vi "get desired labview version.vi"(11 "command line arguments":T1) -> (1 "exe path":path, 2 "lv path specified":bool, 3 "lv version":dbl)   [LabVIEW 2019]
uses:
  arguments.ctl
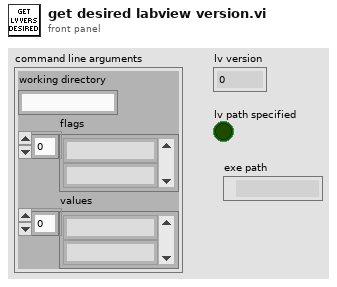
[diagram p1: front panel]
types:
  T1 = typedef "arguments.ctl" = cluster{"working directory":string, "flags":string[], "values":string[]}
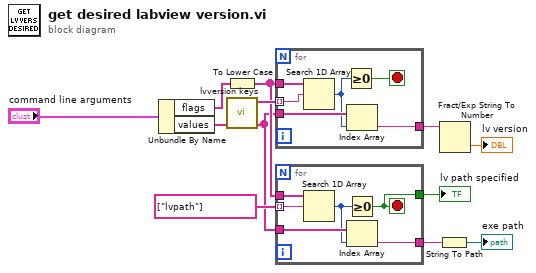
[diagram p0: block diagram]
diagram:
  n1 = Unbundle By Name("command line arguments") -> ("flags"=w7:string[], "values"=w4:string[])
  n2 = To Lower Case(string=w7) -> (all lower case string=w6:string[])
  n3 = call "lvversion keys.vi"() -> ("lv version keys"=w9:string[])  [unwired: 11 in]
  n4 = for {
    tunnel: w6 -> [w17]
    tunnel: w4 -> [w15]
    tunnel: w9 -> [w16] mode=indexing
    tunnel: [w14] -> w8
    stop <- w12 stop-if-true
    n5 = Search 1D Array(1D array=w17, element=w16) -> (index of element=w13:i32)  [unwired: 1 in]
    n6 = Greater Or Equal To 0?(x=w13) -> (x >= 0?=w12:bool)
    n7 = Index Array(array=w15, index=w13) -> (element=w14:string)
  }
  n8 = for {
    tunnel: w6 -> [w23]
    tunnel: w4 -> [w21]
    tunnel: string[] ["lvpath"] ("lv version keys") -> [w22] mode=indexing
    tunnel: [w20] -> w3
    tunnel: [w18] -> w1
    stop <- w18 stop-if-true
    n9 = Search 1D Array(1D array=w23, element=w22) -> (index of element=w19:i32)  [unwired: 1 in]
    n10 = Greater Or Equal To 0?(x=w19) -> (x >= 0?=w18:bool)
    n11 = Index Array(array=w21, index=w19) -> (element=w20:string)
  }
  "lv path specified" <- w1
  n12 = String To Path(string=w3) -> (path=→"exe path":path)
  n13 = Fract/Exp String To Number(string=w8) -> (number=→"lv version":dbl)  [unwired: 3 in, 1 out]
